vi "XLDateToLvDate.vi"(3 "Error In":errorcluster, 4 "XLTimeIn":string[](array[string])=["0.59508932", "0.56268001"], 5 "XLDateIn":string[](array[string])=["40826", "40863"]) -> (0 "Error Out":errorcluster[](array[cluster]), 1 "TimeOut":string[](array[string])=["2:16:56 PM", "1:30:16 PM"], 2 "DateOut":string[](array[string])=["10/10/2011", "11/16/2011"])   [LabVIEW 2012]
doc: "This takes in date and time data from Excel format numbers and calculates it into a normal date and time stamp that can be used in Labview or a report. It ignores daylight savings time by reading it in UTC format."
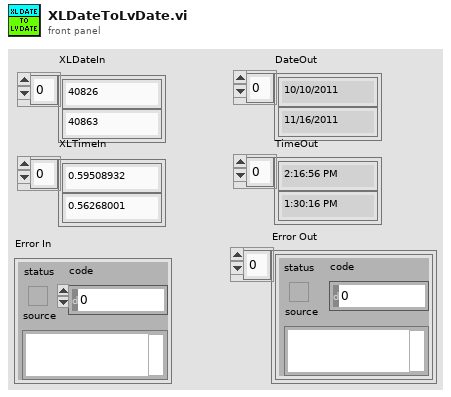
[diagram p1: front panel]
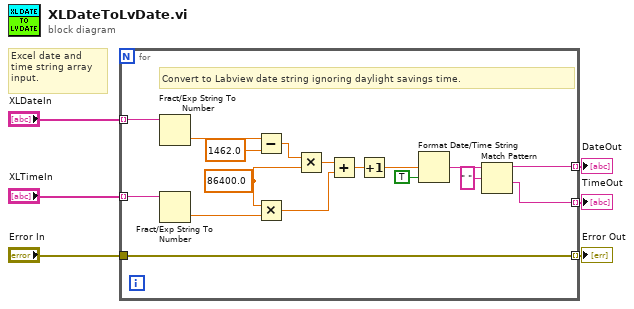
[diagram p0: block diagram]
diagram:
  # "Excel date and time string array input."
  n1 = for {
    tunnel: [w11] -> w4 mode=indexing
    tunnel: [w10] -> w3 mode=indexing
    tunnel: "XLDateIn" -> [w9] mode=indexing
    tunnel: "XLTimeIn" -> [w8] mode=indexing
    tunnel: "Error In" -> [w7]
    tunnel: [w7] -> w1 mode=indexing
    w20 = 86400.0 ("DayToSec")
    # "Convert to Labview date string ignoring daylight savings time."
    n2 = Fract/Exp String To Number(string=w9) -> (number=w21:dbl)  [unwired: 3 in, 1 out]
    n3 = Fract/Exp String To Number(string=w8) -> (number=w19:dbl)  [unwired: 3 in, 1 out]
    n4 = Subtract(x=w21, y=1462.0 ("DateAdj")) -> (x-y=w18:dbl)
    n5 = Multiply(x=w20, y=w19) -> (x*y=w15:dbl)
    n6 = Multiply(x=w18, y=w20) -> (x*y=w23:dbl)
    n7 = Add(x=w23, y=w15) -> (x+y=w14:dbl)
    n8 = Increment(x=w14) -> (x+1=w17:dbl)
    n9 = Format Date/Time String(seconds (now)=w17, UTC format=TRUE) -> (date/time string=w13:string)  [unwired: 1 in]
    n10 = Match Pattern(string=w13, regular expression=" ") -> (before substring=w11:string, after substring=w10:string)  [unwired: 1 in, 2 out]
  }
  "DateOut" <- w4
  "TimeOut" <- w3
  "Error Out" <- w1
